vi "Apply Library Icon to VI.vi"(8 "error in":errorcluster, 11 "VI Reference":refnum<vi>) -> (0 "error out":errorcluster)   [LabVIEW 2020]
doc: "<add documentation>"
uses:
  <vilib>/LabVIEW Icon API/LabVIEW Icon API.lvlib
  C:/Users/Petru/Documents/LabVIEW Data/PopupMenus/edit time panel and diagram/Templates/Target Library/Target Library.lvlib
  <vilib>/LabVIEW Icon API/lv_icon/Classes/Icon/Icon.lvclass
  <vilib>/LabVIEW Icon API/lv_icon/Classes/Icon Framework/Icon Framework.lvclass
  <vilib>/LabVIEW Icon API/lv_icon/Classes/Layer/Layer.lvclass
panel:
  out "User Layer":refnum<class "Layer.lvclass">[](array[class])
  out "VI Icon (after)":picture
  out "VI Icon (before)":picture
  out "Library Icon":picture
  # "Development\ncontrols/indicators useful for development and testing, but which are not outputs of the VI"
  # "Input\nInputs to the VI"
  # "Output\nOutputs of the VI"
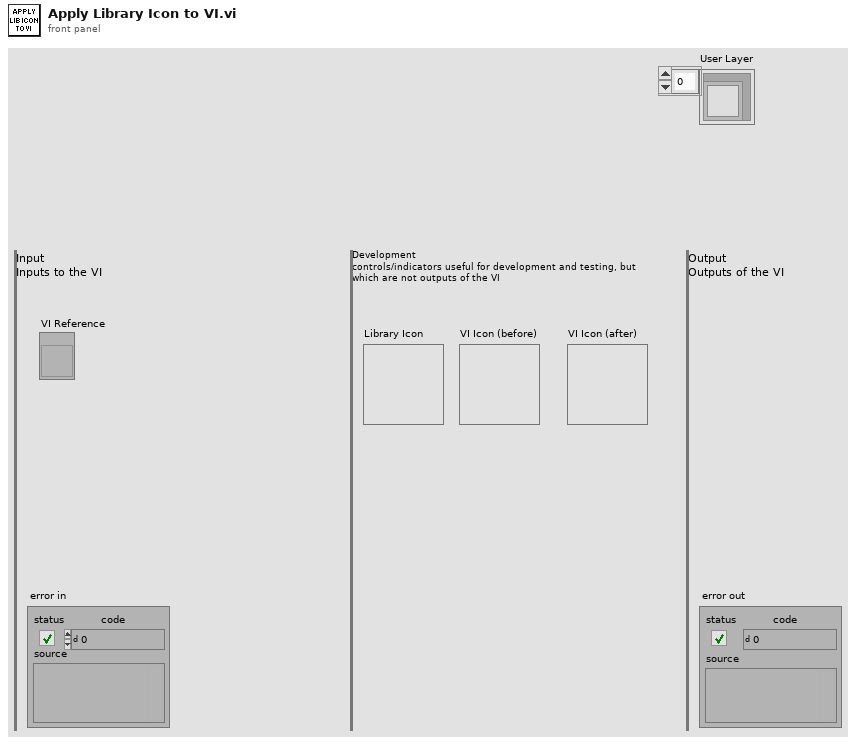
[diagram p1: front panel]
types:
  T1 = typedef "BodyText.ctl" = cluster{"Line 1 text":string, "Line 2 text":string, "Line 3 text":string, "Line 4 text":string, "Line 1 color":u32, "Line 2 color":u32, "Line 3 color":u32, "Line 4 color":u32, "Body Text Spec":cluster{"Font":T2, "Alignment":T3, "Size":u8}, "Center text vertically":bool, "Capitalize Text":bool}
  T2 = typedef "Font.ctl" = string
  T3 = typedef "Alignment.ctl" = u16
  T4 = typedef "imagedata.ctl" = cluster{"image type":i32, "image depth":i32, "image":u8[], "mask":u8[], "colors":u32[], "Rectangle":cluster{"left":i16, "top":i16, "right":i16, "bottom":i16}}
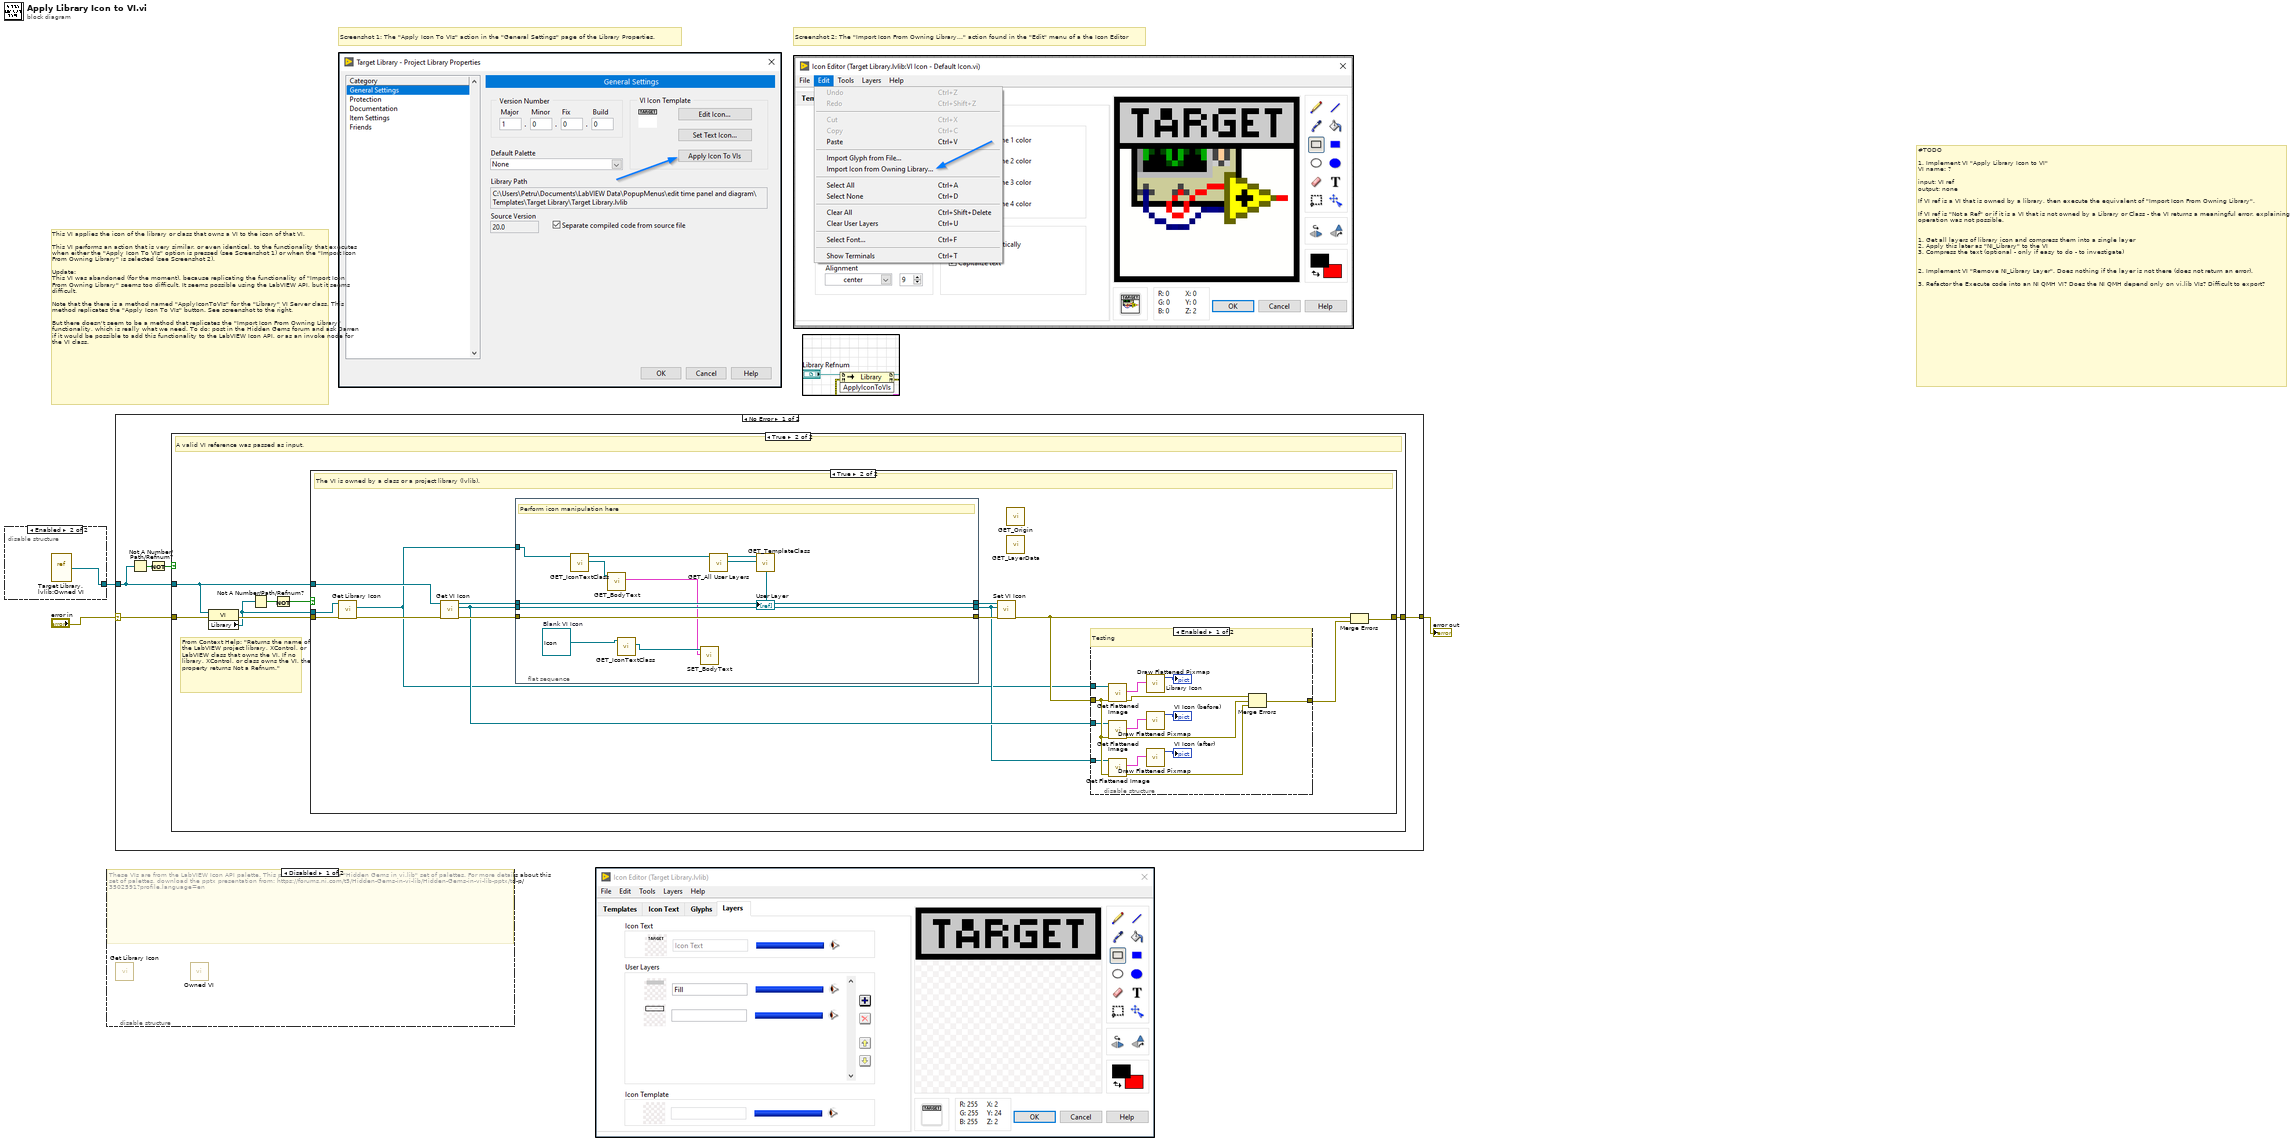
[diagram p0: block diagram]
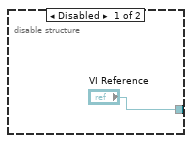
[diagram p2: hidden frame]
diagram:
  # "Screenshot 2: The \"Import Icon From Owning Library...\" action found in the \"Edit\" menu of a the Icon Editor"
  # "Screenshot 1: The \"Apply Icon To VIs\" action in the \"General Settings\" page of the Library Properties."
  # "#TODO\n\n1. Implement VI \"Apply Library Icon to VI\"\nVI name: ?\n\ninput: VI ref\noutput: none\n\nIf VI ref is a VI that is owned by a library, then execute the equivalent of \"Import Icon From Owning Library\".\n\nIf VI ref is \"Not a Ref\" or if it is a VI that is not owned by a Library or Class - the VI returns a meaningful error, explaining that the operation was not possible.\n\n\n1. Get all layers of library icon and compress them into a single layer\n2. Apply this later as \"NI_Library\" to the VI\n3. Compress the text (optional - only if easy to do - to investigate)\n\n\n2. Implement VI \"Remove NI_Library Layer\". Does nothing if the layer is not there (does not return an error).\n\n3. Refactor the Execute code into an NI QMH VI? Does the NI QMH depend only on vi.lib VIs? Difficult to export?"
  # "This VI applies the icon of the library or class that owns a VI to the icon of that VI.\n\nThis VI performs an action that is very similar, or even identical, to the functionality that executes when either the \"Apply Icon To VIs\" option is pressed (see Screenshot 1) or when the \"Import Icon From Owning Library\" is selected (see Screenshot 2).\n\nUpdate:\nThis VI was abandoned (for the moment), because replicating the functionality of \"Import Icon From Owning Library\" seems too difficult. It seems possible using the LabVIEW API, but it seems difficult.\n\nNote that the there is a method named \"ApplyIconToVIs\" for the \"Library\" VI Server class. This method replicates the \"Apply Icon To VIs\" button. See screenshot to the right.\n\nBut there doesn't seem to be a method that replicates the \"Import Icon From Owning Library\" functionality, which is really what we need. To do: post in the Hidden Gems forum and ask Darren if it would be possible to add this functionality to the LabVIEW Icon API, or as an invoke node for the VI class."
  n1 = disable-structure shown="Enabled" {
    disable-tunnel: ["VI Reference" w5] -> w2
    frame Disabled {
    }
    frame Enabled {
      n2 = vi-ref "Target Library.lvlib:Owned VI.vi"() -> (w5:refnum<vi>)
    }
  }
  n3 = disable-structure shown="Disabled" {
    frame Disabled {
      # "These VIs are from the LabVIEW Icon API palette. This palette is part of the \"Hidden Gems in vi.lib\" set of palettes. For more details about this set of palettes, download the pptx presentation from: https://forums.ni.com/t5/Hidden-Gems-in-vi-lib/Hidden-Gems-in-vi-lib-pptx/td-p/3502591?profile.language=en"
      n4 = call <vilib>:"Get Library Icon.vi"() -> ()  [unwired: 9 in, 3 out]
      n5 = call "Owned VI.vi"() -> ()  [unwired: 12 in]
    }
    frame Enabled {
    }
  }
  n6 = case shown="No Error" "error in" {
    selector: "error in" -> [w10 w60]
    tunnel: [w9 w60] -> w1
    tunnel: w2 -> [w8 _]
    frame No Error {
      n7 = Not A Number/Path/Refnum?(number/path/refnum=w8) -> (NaN/Path/Refnum?=w7:bool)
      n8 = Not(x=w7) -> (.not. x?=w6:bool)
      n9 = case shown="True" w6 {
        tunnel: w10 -> [w11 w18]
        tunnel: [w11 w14] -> w9
        tunnel: w8 -> [_ w12]
        frame False {
          # "Do nothing."
          # "Invalid reference at input"
        }
        frame True {
          # "From Context Help: \"Returns the name of the LabVIEW project library, XControl, or LabVIEW class that owns the VI. If no library, XControl, or class owns the VI, the property returns Not a Refnum.\""
          # "A valid VI reference was passed as input."
          n10 = property class="VI"(reference=w12, error in=w18) -> (error out=w15:errorcluster, "Library"=w13:refnum<vi>)  [unwired: 1 out]
          n11 = Not A Number/Path/Refnum?(number/path/refnum=w13) -> (NaN/Path/Refnum?=w17:bool)
          n12 = Not(x=w17) -> (.not. x?=w16:bool)
          n13 = case shown="True" w16 {
            tunnel: w13 -> [_ w32]
            tunnel: w15 -> [w19 w33]
            tunnel: [w19 w30] -> w14
            tunnel: w12 -> [_ w21]
            frame False {
              # "Do nothing."
              # "The VI is not owned by a class or a library"
            }
            frame True {
              # "The VI is owned by a class or a project library (lvlib)."
              n14 = call <vilib>:"Get Library Icon.vi"("error in (no error)"=w33, "Library Refnum in"=w32) -> ("error out"=w31:errorcluster, "Icon"=w20:refnum<class "Icon.lvclass">)  [unwired: 7 in, 1 out]
              n15 = call <vilib>:"Get VI Icon.vi"("error in (no error)"=w31, "VI Refnum in"=w21) -> ("error out"=w27:errorcluster, "Icon"=w23:refnum<class "Icon.lvclass">, "VI Refnum out"=w24:refnum<vi>)  [unwired: 7 in]
              n16 = flat-sequence {
                tunnel: w27 -> [w44]
                tunnel: [w44] -> w26
                tunnel: [w43] -> w25
                tunnel: w24 -> [w43]
                tunnel: w23 -> [w41]
                tunnel: [w41] -> w22
                tunnel: w20 -> [w42]
                frame #0 {
                  w39 = refnum<class "Icon.lvclass"> refnum  # Blank VI Icon
                  # "Perform icon manipulation here"
                  n17 = call-dynamic "GET_IconTextClass.vi"("Icon.lvclass in"=w42) -> ("Icon Framework.lvclass"=w40:refnum<class "Icon Framework.lvclass">, "Icon.lvclass out"=w36:refnum<class "Icon.lvclass">)  [unwired: 8 in, 1 out]
                  n18 = call-dynamic "GET_BodyText.vi"("Icon Framework.lvclass in"=w40) -> ("Body Text"=w37:T1)  [unwired: 7 in, 3 out]
                  n19 = call-dynamic "GET_IconTextClass.vi"("Icon.lvclass in"=w39) -> ("Icon Framework.lvclass"=w38:refnum<class "Icon Framework.lvclass">)  [unwired: 8 in, 2 out]
                  n20 = call-dynamic "SET_BodyText.vi"("Body Text"=w37, "Icon Framework.lvclass in"=w38) -> ()  [unwired: 8 in, 2 out]
                  n21 = call-dynamic "GET_All User Layers.vi"("Icon.lvclass in"=w36) -> ("User Layer"=→"User Layer":refnum<class "Layer.lvclass">[], "Icon.lvclass out"=w35:refnum<class "Icon.lvclass">)  [unwired: 8 in, 1 out]
                  n22 = call-dynamic "GET_TemplateClass.vi"("Icon.lvclass in"=w35) -> ()  [unwired: 8 in, 3 out]
                }
              }
              n23 = call <vilib>:"Set VI Icon.vi"("error in (no error)"=w26, "Icon"=w22, "VI Refnum in"=w25) -> ("error out"=w29:errorcluster)  [unwired: 7 in, 1 out]
              n24 = call-dynamic "GET_Origin.vi"() -> ()  [unwired: 9 in, 3 out]
              n25 = call-dynamic "GET_LayerData.vi"() -> ()  [unwired: 7 in, 5 out]
              n26 = disable-structure shown="Enabled" {
                disable-tunnel: w20 -> [w57 _]
                disable-tunnel: w29 -> [w51 w59]
                disable-tunnel: [w47 w59] -> w28
                disable-tunnel: w23 -> [w46 _]
                disable-tunnel: w22 -> [w45 _]
                frame Enabled {
                  # "Testing"
                  n27 = call <vilib>:"Get Flattened Image.vi"("error in (no error)"=w51, "lv_icon.lvlib:Icon.lvclass in"=w57) -> ("error out"=w50:errorcluster, "Color Image"=w56:T4)  [unwired: 6 in, 2 out]
                  n28 = call <vilib>:"Get Flattened Image.vi"("error in (no error)"=w51, "lv_icon.lvlib:Icon.lvclass in"=w46) -> ("error out"=w49:errorcluster, "Color Image"=w55:T4)  [unwired: 6 in, 2 out]
                  n29 = call <vilib>:"Get Flattened Image.vi"("error in (no error)"=w51, "lv_icon.lvlib:Icon.lvclass in"=w45) -> ("error out"=w48:errorcluster, "Color Image"=w52:T4)  [unwired: 6 in, 2 out]
                  n30 = call <vilib>:"Draw Flattened Pixmap.vi"("image data"=w56) -> ("new picture"=→"Library Icon":picture)  [unwired: 8 in]
                  n31 = call <vilib>:"Draw Flattened Pixmap.vi"("image data"=w55) -> ("new picture"=→"VI Icon (before)":picture)  [unwired: 8 in]
                  n32 = call <vilib>:"Draw Flattened Pixmap.vi"("image data"=w52) -> ("new picture"=→"VI Icon (after)":picture)  [unwired: 8 in]
                  n33 = Merge Errors(w50, w49, w48) -> (w47:errorcluster)
                }
                frame Disabled {
                  # "Production Code"
                }
              }
              n34 = Merge Errors(w29, w28) -> (w30:errorcluster)
            }
          }
        }
      }
    }
    frame Error {
    }
  }
  "error out" <- w1
